vi "SFP.vi"(0 "sfp 0.resources":T2, 5 "sfp 1.resources":T1) -> ()   [LabVIEW 2016]
uses:
  <instrlib>/_niInstr/CLIP Adapters/v1/FPGA/AXI4-Stream/Writer FXP64x1/niInstr AXI4-Stream Writer FXP64x1 v1 FPGA.lvclass
  <instrlib>/_niInstr/CLIP Adapters/v1/FPGA/AXI4-Stream/Reader FXP64x1/niInstr AXI4-Stream Reader FXP64x1 v1 FPGA.lvclass
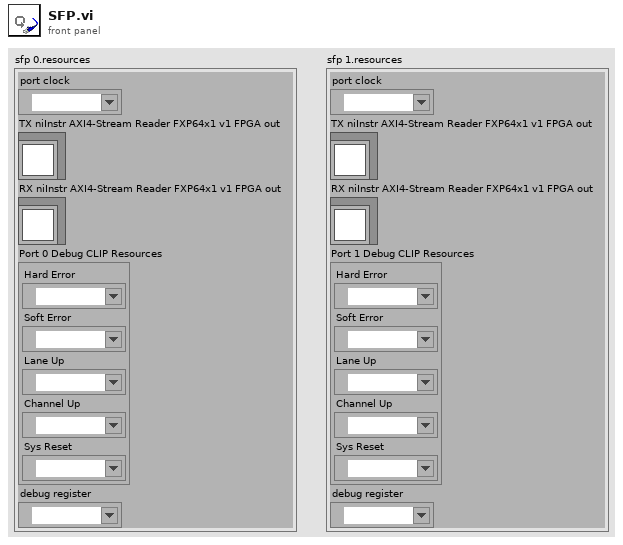
[diagram p1: front panel]
types:
  T1 = cluster{"port clock":refnum<k21>, "TX niInstr AXI4-Stream Reader FXP64x1 v1 FPGA out":refnum<class "niInstr AXI4-Stream Writer FXP64x1 v1 FPGA.lvclass">, "RX niInstr AXI4-Stream Reader FXP64x1 v1 FPGA out":refnum<class "niInstr AXI4-Stream Reader FXP64x1 v1 FPGA.lvclass">, "Port 1 Debug CLIP Resources":cluster{"Hard Error":refnum<k21>, "Soft Error":refnum<k21>, "Lane Up":refnum<k21>, "Channel Up":refnum<k21>, "Sys Reset":refnum<k21>}, "debug register":refnum<k21>}
  T2 = cluster{"port clock":refnum<k21>, "TX niInstr AXI4-Stream Reader FXP64x1 v1 FPGA out":refnum<class "niInstr AXI4-Stream Writer FXP64x1 v1 FPGA.lvclass">, "RX niInstr AXI4-Stream Reader FXP64x1 v1 FPGA out":refnum<class "niInstr AXI4-Stream Reader FXP64x1 v1 FPGA.lvclass">, "Port 0 Debug CLIP Resources":cluster{"Hard Error":refnum<k21>, "Soft Error":refnum<k21>, "Lane Up":refnum<k21>, "Channel Up":refnum<k21>, "Sys Reset":refnum<k21>}, "debug register":refnum<k21>}
  T3 = cluster{"Hard Error":refnum<k21>, "Soft Error":refnum<k21>, "Lane Up":refnum<k21>, "Channel Up":refnum<k21>, "Sys Reset":refnum<k21>}
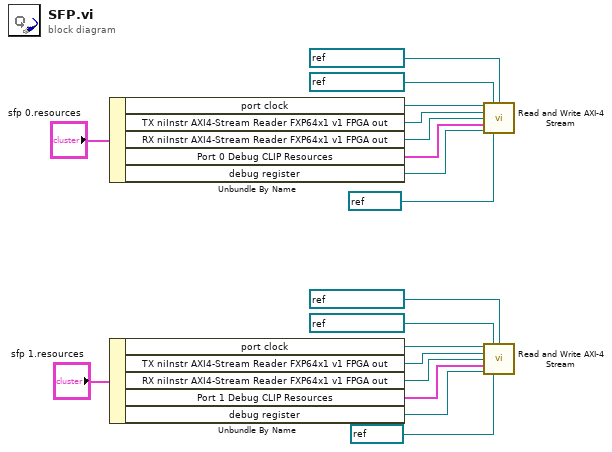
[diagram p0: block diagram]
diagram:
  n1 = Unbundle By Name("sfp 0.resources") -> ("port clock"=w14:refnum<k21>, "TX niInstr AXI4-Stream Reader FXP64x1 v1 FPGA out"=w13:refnum<class "niInstr AXI4-Stream Writer FXP64x1 v1 FPGA.lvclass">, "RX niInstr AXI4-Stream Reader FXP64x1 v1 FPGA out"=w12:refnum<class "niInstr AXI4-Stream Reader FXP64x1 v1 FPGA.lvclass">, "Port 0 Debug CLIP Resources"=w11:T3, "debug register"=w10:refnum<k21>)
  n2 = Unbundle By Name("sfp 1.resources") -> ("port clock"=w8:refnum<k21>, "TX niInstr AXI4-Stream Reader FXP64x1 v1 FPGA out"=w6:refnum<class "niInstr AXI4-Stream Writer FXP64x1 v1 FPGA.lvclass">, "RX niInstr AXI4-Stream Reader FXP64x1 v1 FPGA out"=w7:refnum<class "niInstr AXI4-Stream Reader FXP64x1 v1 FPGA.lvclass">, "Port 1 Debug CLIP Resources"=w5:T3, "debug register"=w4:refnum<k21>)
  n3 = call "Read and Write AXI-4 Stream.vi"("port clock"=w14, "rx 0.sfp fifo"=refnum<k21> "rx 0.sfp 0 fifo" ("FIFO"), "rx 1.sfp fifo"=refnum<k21> "rx 1.sfp 0 fifo" ("FIFO"), "TX niInstr AXI4-Stream Reader FXP64x1 v1 FPGA out"=w13, "RX niInstr AXI4-Stream Reader FXP64x1 v1 FPGA out"=w12, "port debug CLIP resources"=w11, "port debug info"=w10, "Register"=refnum<k21> "SFP0") -> ()  [unwired: 8 in]
  n4 = call "Read and Write AXI-4 Stream.vi"("port clock"=w8, "rx 0.sfp fifo"=refnum<k21> "rx 2.sfp 1 fifo" ("FIFO"), "rx 1.sfp fifo"=refnum<k21> "rx 3.sfp 1 fifo" ("FIFO"), "TX niInstr AXI4-Stream Reader FXP64x1 v1 FPGA out"=w6, "RX niInstr AXI4-Stream Reader FXP64x1 v1 FPGA out"=w7, "port debug CLIP resources"=w5, "port debug info"=w4, "Register"=refnum<k21> "SFP1") -> ()  [unwired: 8 in]
